vi "test Get-Set-Get Description.vi"(8 "error in":errorcluster, 11 "TestCase in":refnum<class "Scripting.lvclass">) -> (0 "error out":errorcluster, 3 "TestCase out":refnum<class "Scripting.lvclass">)   [LabVIEW 2020, in "Scripting.lvclass"]
uses:
  Scripting.lvclass
  <vilib>/addons/_JKI Toolkits/VI Tester/TestCase.llb/TestCase.lvclass
  Scripting/Ballard MIL-STD-1553 Scripting.lvlib
  C:/Git/niveristand-custom-device-testing-tools/VeriStandScriptingTestCase/VeriStandScriptingTestCase.lvclass
  C:/Program Files (x86)/National Instruments/LabVIEW 2020/vi.lib/addons/_JKI Toolkits/VI Tester/TestCase.llb/TestCase.lvclass
  C:/Git/niveristand-ballard-milStd1553-custom-device/Source/Custom Device Support/Tests/Unit/Scripting/Scripting.lvclass
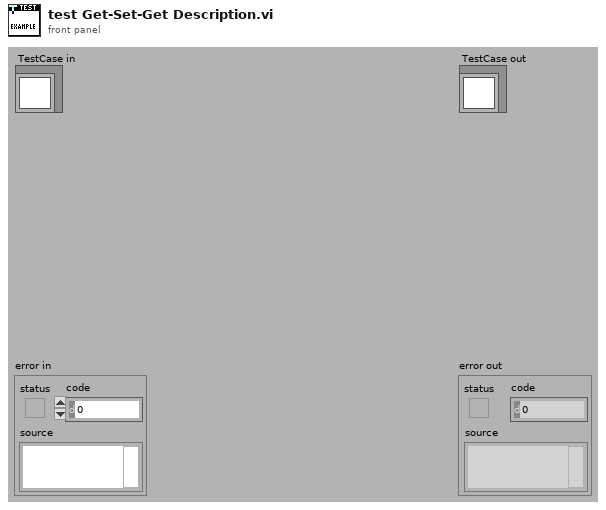
[diagram p1: front panel]
types:
  T1 = typedef "Custom Device API.lvlib/Custom Device Item Ref.ctl" = u64
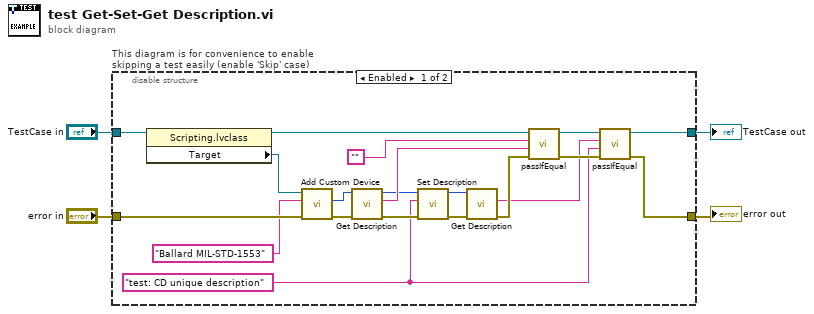
[diagram p0: block diagram]
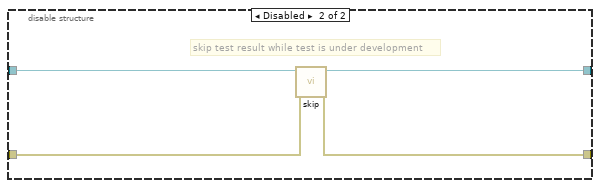
[diagram p2: hidden frame]
diagram:
  n1 = disable-structure "This diagram is for convenience to enable skipping a test easily (enable 'Skip' case)" shown="Enabled" {
    disable-tunnel: "TestCase in" -> [w20 w28]
    disable-tunnel: [w22 w26] -> w1
    disable-tunnel: [w21 w27] -> w3
    disable-tunnel: "error in" -> [w24 w25]
    frame Enabled {
      w5 = "test: CD unique description" ("name")
      n2 = property class="Scripting.lvclass"(reference=w20) -> (reference out=w18:refnum<class "Scripting.lvclass">, "Target"=w19:refnum<k24>)  [unwired: 1 in, 1 out]
      n3 = call "Add Custom Device.vi"("error in"=w24, "name"="Ballard MIL-STD-1553", "target in"=w19) -> ("error out"=w17:errorcluster, "Ballard MIL-STD 1553 custom device"=w16:T1)  [unwired: 6 in, 1 out]
      n4 = call "Get Description.vi"("error in"=w17, "Ballard MIL-STD 1553 custom device in"=w16) -> ("error out"=w12:errorcluster, "description"=w15:string, "Ballard MIL-STD 1553 custom device out"=w13:T1)  [unwired: 7 in]
      n5 = call "Set Description.vi"("error in"=w12, "description"=w5, "Ballard MIL-STD 1553 custom device in"=w13) -> ("error out"=w11:errorcluster, "Ballard MIL-STD 1553 custom device out"=w10:T1)  [unwired: 7 in]
      n6 = call "Get Description.vi"("error in"=w11, "Ballard MIL-STD 1553 custom device in"=w10) -> ("error out"=w9:errorcluster, "description"=w6:string)  [unwired: 7 in, 1 out]
      n7 = call-dynamic "passIfEqual.vi"("error in (no error)"=w9, "y"=w15, "x"="", "TestCase in"=w18) -> ("error out"=w7:errorcluster, "TestCase out"=w8:refnum<class "Scripting.lvclass">)  [unwired: 6 in]
      n8 = call-dynamic "passIfEqual.vi"("error in (no error)"=w7, "y"=w5, "x"=w6, "TestCase in"=w8) -> ("error out"=w21:errorcluster, "TestCase out"=w22:refnum<class "Scripting.lvclass">)  [unwired: 6 in]
    }
    frame Disabled {
      # "skip test result while test is under development"
      n9 = call <vilib>:"skip.vi"("error in (no error)"=w25, "TestCase in"=w28) -> ("error out"=w27:errorcluster, "TestCase out"=w26:refnum<class "Scripting.lvclass">)  [unwired: 8 in]
    }
  }
  "error out" <- w3
  "TestCase out" <- w1
